vi "Filter Banks - 1D.vi"() -> ()   [LabVIEW 2023]
doc: "This example shows how to acquire the detail coefficients and the approximation coefficients of a signal with the WA Analysis Filter Bank VI. This example also shows how to reconstruct the signal from the detail coefficients and the approximation coefficients with the WA Synthesis Filter Bank VI.\n\n<b>Instructions:</b>\n1) Run this VI.\n2) Observe the <b>Detail Coefficients</b> and the <b>Approximation Coefficients</b> of the <b>Signal</b>.\n3) Browse the Block Diagram to learn how to use the WA Analysis Filter Bank VI to perform one-level decomposition on a signal, how to use the WA Synthesis Filter Bank VI to reconstruct the signal, and how to use the WA Wavelet Filter VI to read analysis filters and synthesis filters of a wavelet."
uses:
  <vilib>/addons/Wavelet Analysis/filter banks.llb/WA 1D Analysis Filter Bank (Waveform).vi
  <vilib>/addons/Wavelet Analysis/filter banks.llb/WA 1D Synthesis Filter Bank (Waveform).vi
  <vilib>/addons/_Advanced Signal Processing/NI_AdvSigProcWA.lvlib
panel:
  in  "Data":u16(ring)=103 items=["1D Example Data"=100, "-"=101, "Doppler"=102, "HOP"=103, "TF Sine"=104, "Noisy Doppler"=105, "Sea Temperature"=106, "Sp500"=107, "Power Line"=108, "Engine Knocking"=109, "HeaviSine"=110, "Bumps"=111, "Blocks"=112, "Piece Regular"=113, "HypChirps"=114, "LinChirps"=115, "Chirps"=116, "Piece Polynomial"=117, "ECG"=131, "-"=118, "2D Example Data"=119, "-"=120, "Finger Print (Image)"=121, "Iris Flower (Image)"=122, "Mammogram (Image)"=123, "Lake (Image)"=127, "Two Can 1 (Image)"=132, "Two Can 2 (Image)"=133, "Camera Man (Image)"=134]
  in  "stop":bool
  out "Detail Coefficients":waveform(dbl)(graph)
  out "Approximation Coefficients":waveform(dbl)(graph)
  out "Signal":waveform(dbl)[](graph)
  in  "Wavelet":u16(ring) items=["db02"=0, "db03"=1, "db04"=2, "db05"=3, "db06"=4, "db07"=5, "db08"=6, "db09"=7, "db10"=8, "db11"=9, "db12"=10, "db13"=11, "db14"=12, "Haar"=13, "bior1_3"=14, "bior1_5"=15, "bior2_2"=16, "bior2_4"=17, "bior2_6"=18, "bior2_8"=19, "bior3_1"=20, "bior3_3"=21, "bior3_5"=22, "bior3_7"=23, "bior3_9"=24, "bior4_4 (FBI)"=25, "bior5_5"=38, "bior6_8"=39, "coif1"=26, "coif2"=27, "coif3"=28, "coif4"=29, "coif5"=30, "sym2"=31, "sym3"=32, "sym4"=33, "sym5"=34, "sym6"=35, "sym7"=36, "sym8"=37]
  in  "Extension":u16(ring)=1 items=["Zero padding", "Symmetric", "Periodic", "Spline"]
  # "Overview: Shows how to acquire the detail coefficients and the approximation coefficients of a signal with the WA Analysis Filter Bank VI. \nRequirements: LabVIEW Full Development System, Advanced Signal Processing Toolkit\nInstructions: \n1. Run this VI.\n2. Observe the Detail Coefficients and the Approximation Coefficients of the Signal.\n3. Browse the block diagram to learn how to use the WA Analysis Filter Bank VI to perform one-level decomposition on a signal, how to use the WA Synthesis Filter Bank VI to reconstruct the signal, and how to use the WA Wavelet Filter VI to read analysis filters and synthesis filters of a wavelet.\n4. Click Stop to stop the VI."
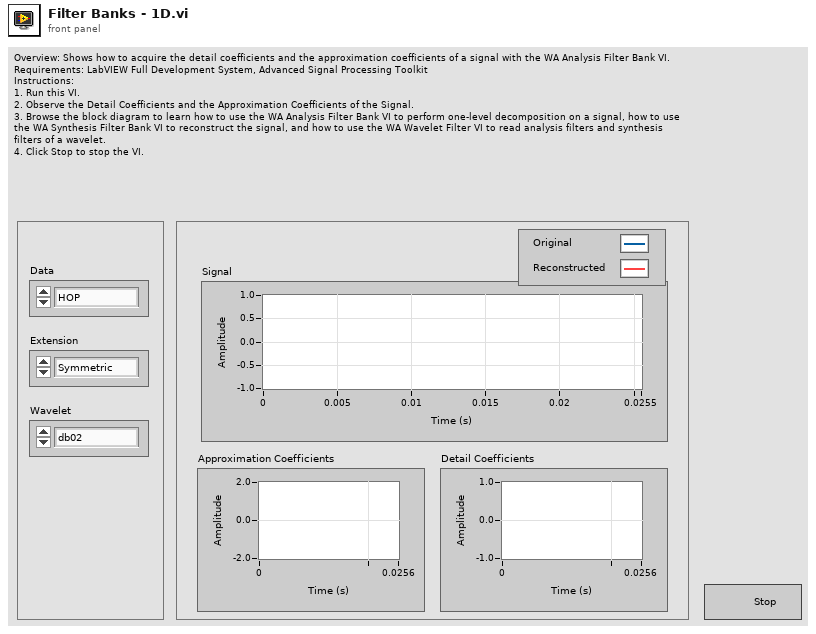
[diagram p1: front panel]
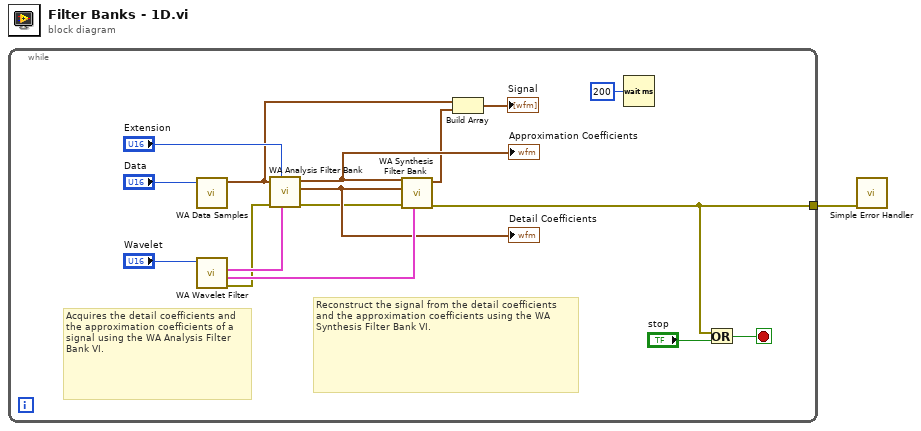
[diagram p0: block diagram]
diagram:
  n1 = while {
    tunnel: [w3] -> w1
    stop <- w6 stop-if-true
    # "Reconstruct the signal from the detail coefficients and the approximation coefficients using the WA Synthesis Filter Bank VI."
    # "Acquires the detail coefficients and the approximation coefficients of a signal using the WA Analysis Filter Bank VI."
    n2 = call <vilib>:"WA Data Samples.vi"("data"="Data") -> ("signal"=w9:waveform(dbl))  [unwired: 10 out]
    n3 = call <vilib>:"WA Wavelet Filter.vi"("wavelet"="Wavelet") -> ("error out"=w2:errorcluster, "synthesis filters"=w15:cluster{"lowpass":dbl[], "highpass":dbl[]}, "analysis filters"=w16:cluster{"lowpass":dbl[], "highpass":dbl[]})  [unwired: 3 in, 5 out]
    n4 = call-poly <vilib>:"WA Analysis Filter Bank.vi"("analysis filters"=w16, "extension"="Extension", "error in (no error)"=w2, "signal"=w9) -> ("error out"=w11:errorcluster, "detail coef"=w12:waveform(dbl), "approx coef"=w13:waveform(dbl))  [unwired: 5 out]
    "Approximation Coefficients" <- w13
    "Detail Coefficients" <- w12
    n5 = call-poly <vilib>:"WA Synthesis Filter Bank.vi"("synthesis filters"=w15, "error in (no error)"=w11, "detail coef"=w12, "approx coef"=w13) -> ("error out"=w3:errorcluster, "signal"=w10:waveform(dbl))  [unwired: 6 out]
    n6 = Build Array(w9, w10) -> (→"Signal":waveform(dbl)[])
    n7 = Wait (ms)(milliseconds to wait=u32 200 ("millisecond multiple")) -> ()  [unwired: 1 out]
    n8 = Or(x=w3, y="stop") -> (x .or. y?=w6:bool)
  }
  n9 = call <vilib>:"Simple Error Handler.vi"("error in (no error)"=w1) -> ()  [unwired: 1 in, 8 out]
